vi "Timestamp Reservations.vi"(3 "Reset":bool, 5 "Line":tag) -> (0 "Exit code":T1, 1 "Index assigned":i32, 2 "DigitalOutput lines":tag[](array[tag]))   [LabVIEW 2015]
doc: "Attempt to reserve a line as a digital output. This also returns a list of lines that have been previously reserved.\n\nAs a Device developer, just call this with the line you want to add, check that the exit code is good, and save the assigned index.\n\nAs a Rack developer, remember to reset the reservations list before Device initialization and then call it with an empty line afterwards to get the list of digital output lines."
uses:
  Typedefs/Reservation exit codes.ctl
  <vilib>/Utility/error.llb/DialogType.ctl
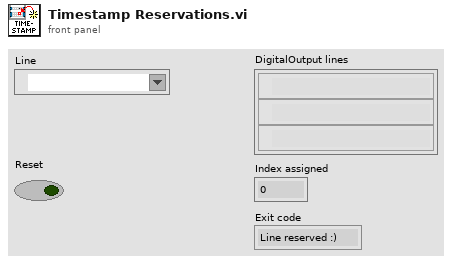
[diagram p1: front panel]
types:
  T1 = typedef "Reservation exit codes.ctl" = enum16{"Line reserved :)", "List reset.", "Empty line!", "Bad line!", "Already reserved!", "Timestamp conflict!", "Timestamp empty."}
  T2 = typedef "DialogType.ctl" = u16
  T3 = enum16{"Analog input", "Analog output", "Digital input", "Digital output", "Counter input", "Counter output"}
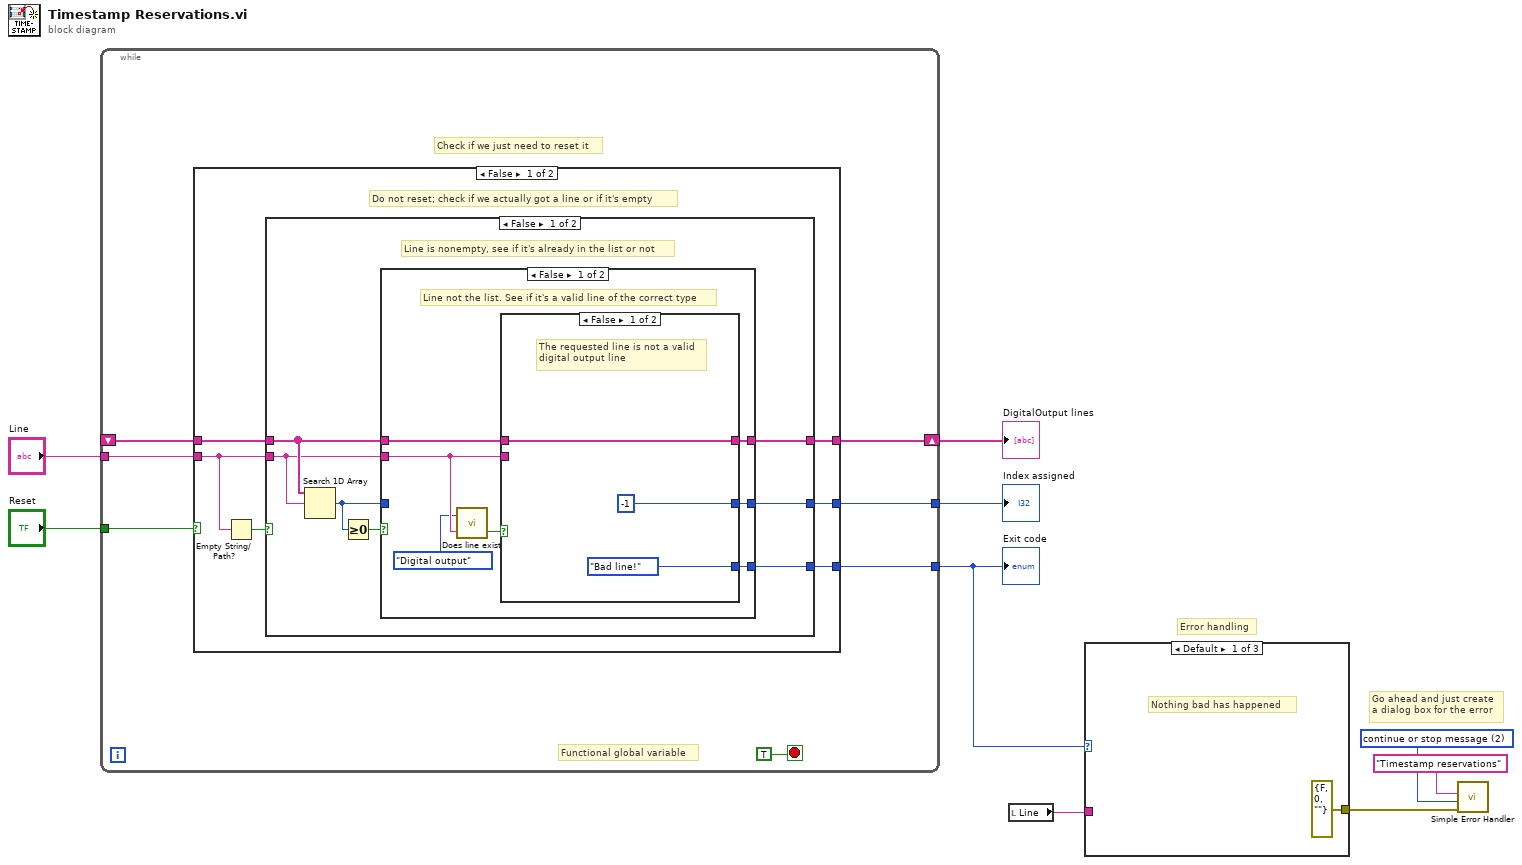
[diagram p0: block diagram]
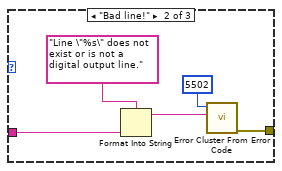
[diagram p2: hidden frame]
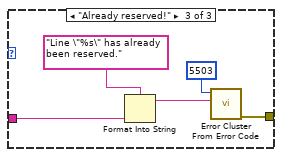
[diagram p3: hidden frame]
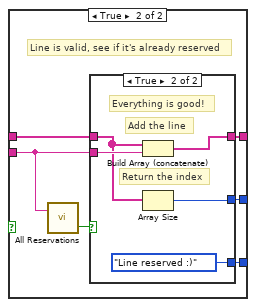
[diagram p4: hidden frame]
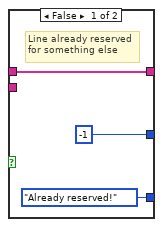
[diagram p5: hidden frame]
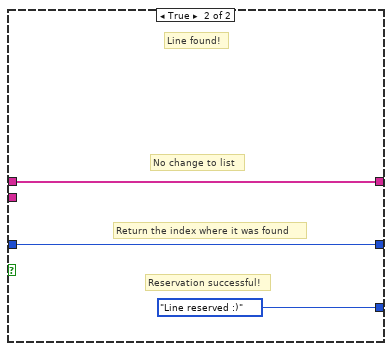
[diagram p6: hidden frame]
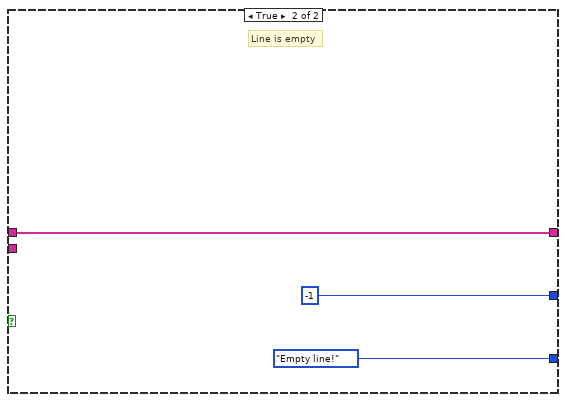
[diagram p7: hidden frame]
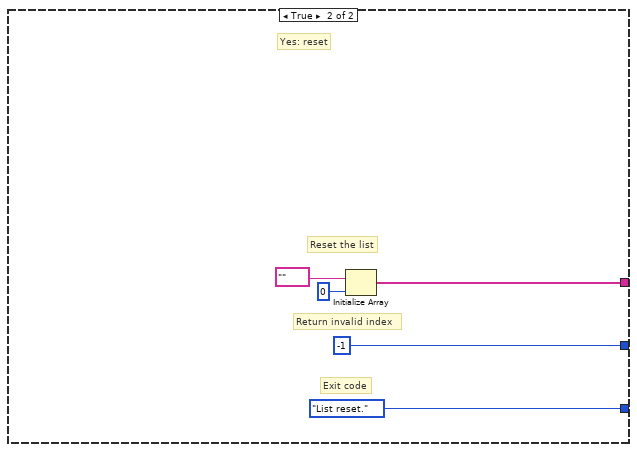
[diagram p8: hidden frame]
diagram:
  w4 = T2 2 items=["no dialog", "OK message", "continue or stop message", "OK message + warnings", "continue/stop + warnings"] ("type of dialog (OK msg:1)")
  # "Error handling"
  # "Go ahead and just create\na dialog box for the error"
  n1 = while {
    tunnel: [w16] -> w6
    tunnel: "Reset" -> [w15]
    shift-right: [w14] -> w9
    shift-left: _ -> [w12]
    tunnel: "Line" -> [w11]
    tunnel: [w10] -> w7
    stop <- TRUE ("stop") stop-if-true
    # "Check if we just need to reset it"
    # "Functional global variable"
    n2 = case shown="False" w15 {
      tunnel: [w19 Reservation_exit_codes."List reset." ("Exit code")] -> w16
      tunnel: [w22 w63] -> w14
      tunnel: w12 -> [w21 _]
      tunnel: w11 -> [w17 _]
      tunnel: [w20 -1 ("Index assigned")] -> w10
      frame False {
        # "Do not reset; check if we actually got a line or if it's empty"
        n3 = Empty String/Path?(string/path=w17) -> (empty?=w18:bool)
        n4 = case shown="False" w18 {
          tunnel: [w29 w59] -> w22
          tunnel: w21 -> [w25 w59]
          tunnel: [w28 -1] -> w20
          tunnel: [w27 Reservation_exit_codes."Empty line!" ("Exit code")] -> w19
          tunnel: w17 -> [w24 _]
          frame False {
            # "Line is nonempty, see if it's already in the list or not"
            n5 = Search 1D Array(1D array=w25, element=w24) -> (index of element=w23:i32)  [unwired: 1 in]
            n6 = Greater Or Equal To 0?(x=w23) -> (x >= 0?=w26:bool)
            n7 = case shown="False" w26 {
              tunnel: [w36 w55] -> w29
              tunnel: w25 -> [w35 w55]
              tunnel: [w34 w56] -> w28
              tunnel: [w33 Reservation_exit_codes."Line reserved :)" ("Exit code")] -> w27
              tunnel: w24 -> [w31 _]
              tunnel: w23 -> [_ w56]
              frame False {
                # "Line not the list. See if it's a valid line of the correct type"
                n8 = call "Does line exist.vi"("Line to look for"=w31, "Line type"=T3."Digital output") -> ("Does line exist?"=w32:bool)  [unwired: 1 out]
                n9 = case shown="False" w32 {
                  tunnel: [w39 w45] -> w36
                  tunnel: w35 -> [w39 w44]
                  tunnel: [-1 w43] -> w34
                  tunnel: [Reservation_exit_codes."Bad line!" ("Exit code") w42] -> w33
                  tunnel: w31 -> [_ w40]
                  frame False {
                    # "The requested line is not a valid\ndigital output line"
                  }
                  frame True {
                    # "Line is valid, see if it's already reserved"
                    n10 = call "All Reservations.vi"("Line to add"=w40) -> ("Line added?"=w41:bool)  [unwired: 1 in, 1 out]
                    n11 = case shown="True" w41 {
                      tunnel: w44 -> [w48 w51]
                      tunnel: [w48 w53] -> w45
                      tunnel: w40 -> [_ w52]
                      tunnel: [-1 w50] -> w43
                      tunnel: [Reservation_exit_codes."Already reserved!" ("Exit code") Reservation_exit_codes."Line reserved :)" ("Exit code")] -> w42
                      frame False {
                        # "Line already reserved\nfor something else"
                      }
                      frame True {
                        # "Everything is good!"
                        # "Return the index"
                        # "Add the line"
                        n12 = Build Array (concatenate)(w51, w52) -> (w53:tag[])
                        n13 = Array Size(array=w51) -> (size(s)=w50:i32)
                      }
                    }
                  }
                }
              }
              frame True {
                # "Reservation successful!"
                # "Return the index where it was found"
                # "No change to list"
                # "Line found!"
              }
            }
          }
          frame True {
            # "Line is empty"
          }
        }
      }
      frame True {
        # "Yes: reset"
        # "Exit code"
        # "Return invalid index"
        # "Reset the list"
        n14 = Initialize Array(tag "" ("Line to add"), 0 ("dimension size")) -> (w63:tag[])
      }
    }
  }
  "DigitalOutput lines" <- w9
  "Exit code" <- w6
  "Index assigned" <- w7
  n15 = local read "Line"() -> (w1:tag)
  n16 = case shown="Default" w6 {
    tunnel: w1 -> [_ w67 w71]
    tunnel: [errorcluster {"status"=FALSE, "code"=0, "source"=""} ("error out") w66 w72] -> w2
    frame Default {
      # "Nothing bad has happened"
    }
    frame "Bad line!" {
      n17 = Format Into String(format string="Line \"%s\" does not exist or is not a digital output line.", w67) -> (resulting string=w70:string)  [unwired: 2 in, 1 out]
      n18 = call <vilib>:"Error Cluster From Error Code.vi"("error message (\"\")"=w70, "error code (0)"=5502) -> ("error out"=w66:errorcluster)  [unwired: 7 in]
    }
    frame "Already reserved!" {
      n19 = Format Into String(format string="Line \"%s\" has already been reserved.", w71) -> (resulting string=w73:string)  [unwired: 2 in, 1 out]
      n20 = call <vilib>:"Error Cluster From Error Code.vi"("error message (\"\")"=w73, "error code (0)"=5503) -> ("error out"=w72:errorcluster)  [unwired: 7 in]
    }
  }
  n21 = call <vilib>:"Simple Error Handler.vi"("error source (\" \")"="Timestamp reservations" ("error source (\" \")"), "type of dialog (OK msg:1)"=w4, "error in (no error)"=w2) -> ()  [unwired: 2 in, 5 out]
